vi "Str_Out.vi"() -> (2 "String_Out":string)   [LabVIEW 2018]
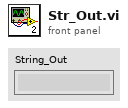
[diagram p1: front panel]
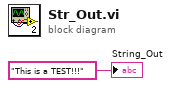
[diagram p0: block diagram]
diagram:
  "String_Out" <- "This is a TEST!!!" ("String_Out")
